vi "producer_consumer queue test.vi"() -> ()   [LabVIEW 2023]
panel:
  in  "Consumer Loop Delay (msec)":u32=2
  in  "Producer loop delay(msec)":u32=2
  out "Queue Output Array":dbl[][](array[numeric])
  out "Test Array":dbl[][](array[numeric])
  out "error out":errorcluster
  in  "error in (no error)":errorcluster
  in  "Queue Status Loop Time(msec)":u32=50
  in  "stop":bool
  out "Elements in Queue":i32
  in  "Max Queue Size":i32=1000
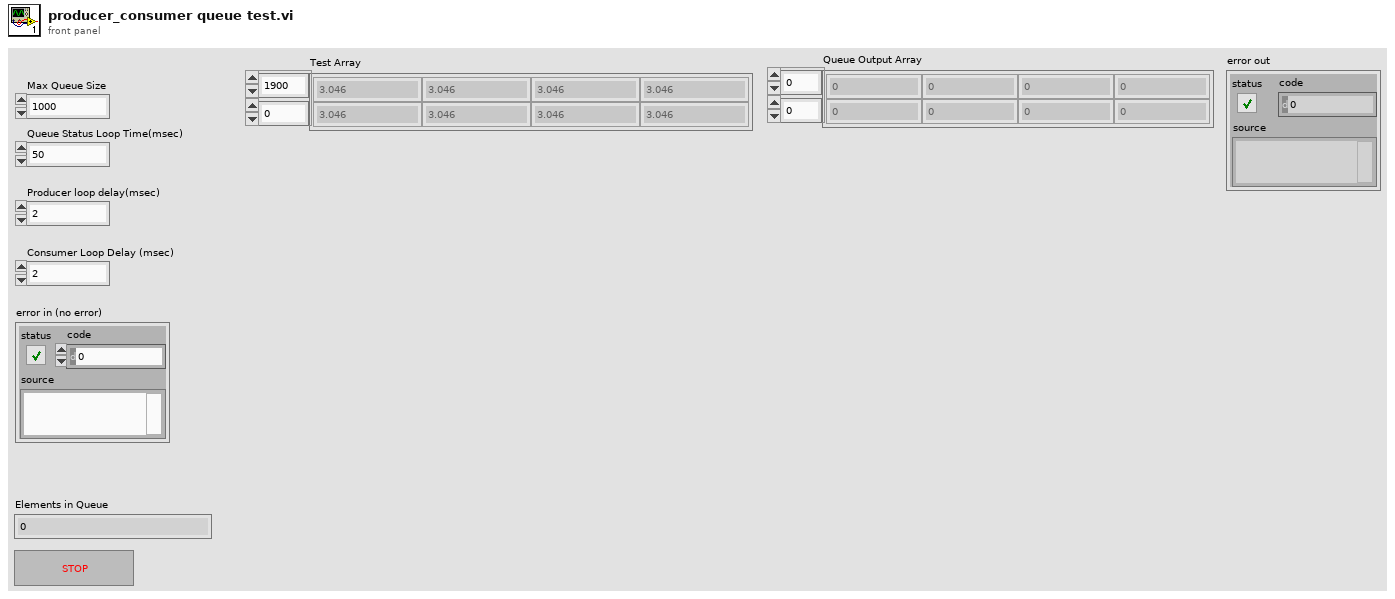
[diagram p1: front panel]
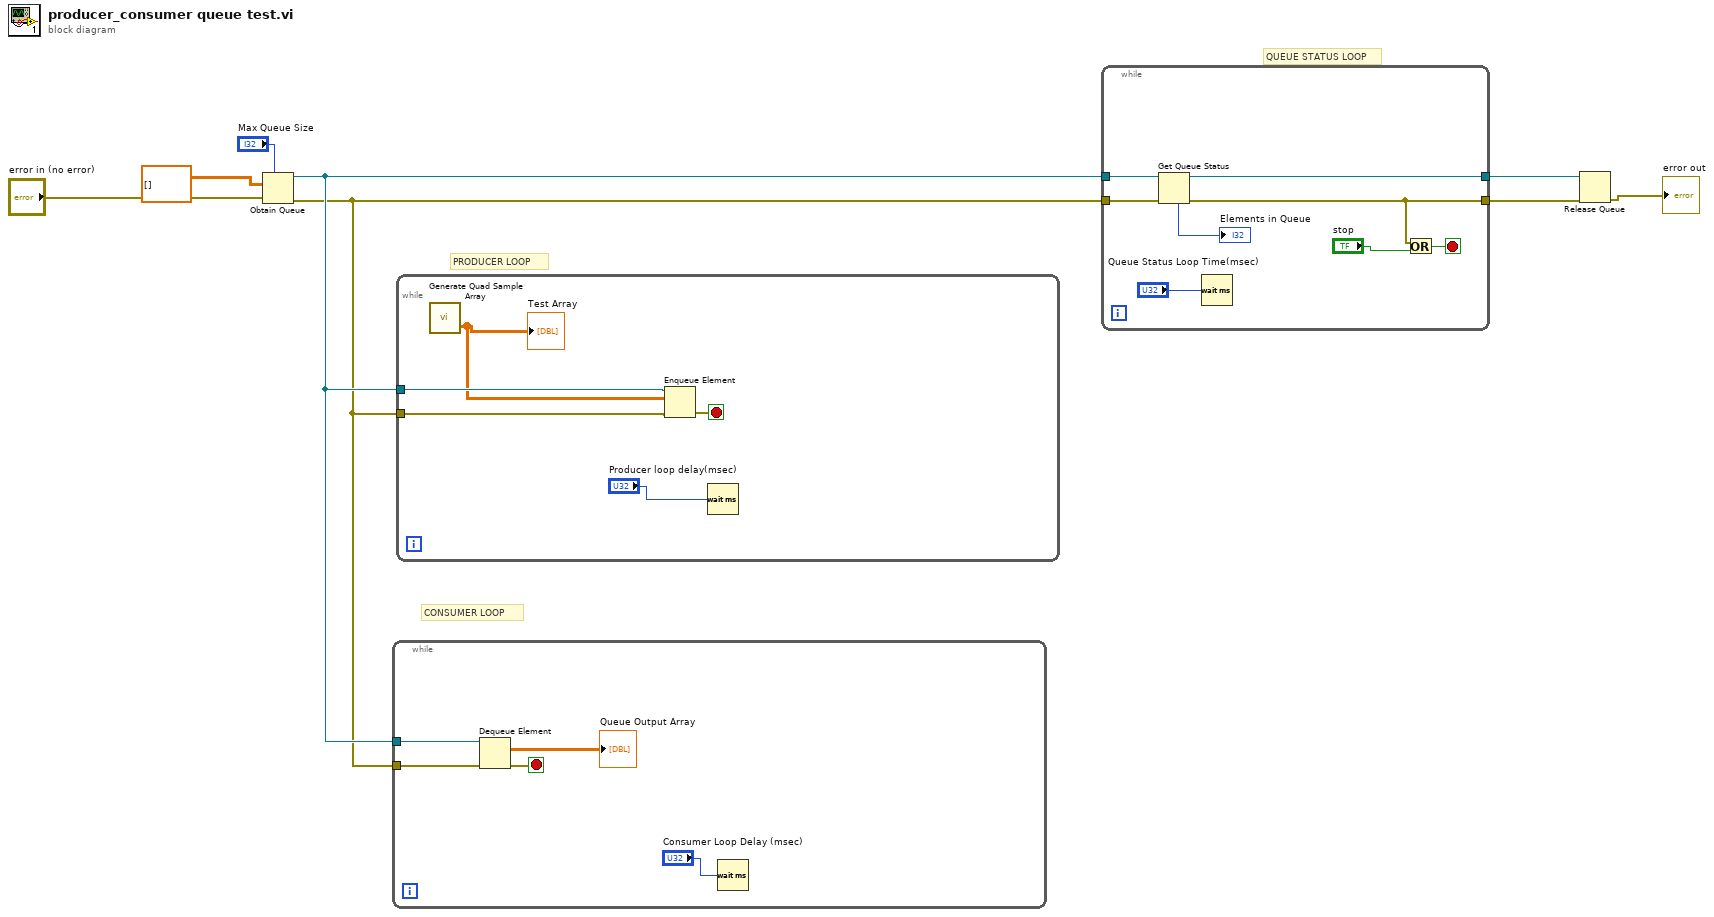
[diagram p0: block diagram]
diagram:
  # "QUEUE STATUS LOOP"
  # "CONSUMER LOOP"
  # "PRODUCER LOOP"
  n1 = Obtain Queue(max queue size (-1, unlimited)="Max Queue Size", element data type=dbl[][] [], error in (no error)="error in (no error)") -> (queue out=w6:refnum<queue>, error out=w5:errorcluster)  [unwired: 2 in, 1 out]
  n2 = while {
    tunnel: w6 -> [w13]
    tunnel: w5 -> [w12]
    stop <- w11 stop-if-true
    n3 = Dequeue Element(queue=w13, error in (no error)=w12) -> (element=→"Queue Output Array":dbl[][], error out=w11:errorcluster)  [unwired: 1 in, 2 out]
    n4 = Wait (ms)(milliseconds to wait="Consumer Loop Delay (msec)") -> ()  [unwired: 1 out]
  }
  n5 = while {
    tunnel: w6 -> [w18]
    tunnel: w5 -> [w17]
    stop <- w16 stop-if-true
    n6 = call "Generate Quad Sample Array.vi"() -> ("Initialized & Randomized 4 x 25 Array"=w14:dbl[][])  [unwired: 5 in]
    "Test Array" <- w14
    n7 = Enqueue Element(queue=w18, element=w14, error in (no error)=w17) -> (error out=w16:errorcluster)  [unwired: 1 in, 2 out]
    n8 = Wait (ms)(milliseconds to wait="Producer loop delay(msec)") -> ()  [unwired: 1 out]
  }
  n9 = while {
    tunnel: w6 -> [w26]
    tunnel: w5 -> [w25]
    tunnel: [w24] -> w8
    tunnel: [w21] -> w7
    stop <- w22 stop-if-true
    n10 = Get Queue Status(queue=w26, error in (no error)=w25) -> (queue out=w24:refnum<queue>, error out=w21:errorcluster, # elements in queue=→"Elements in Queue":i32)  [unwired: 1 in, 5 out]
    n11 = Wait (ms)(milliseconds to wait="Queue Status Loop Time(msec)") -> ()  [unwired: 1 out]
    n12 = Or(x=w21, y="stop") -> (x .or. y?=w22:bool)
  }
  n13 = Release Queue(queue=w8, error in (no error)=w7) -> (error out=→"error out":errorcluster)  [unwired: 1 in, 2 out]
